vi "read_pelletronV1.vi"(8 "error in (no error)":errorcluster, 10 "Lower Timestamp Limit":i64, 11 "Upper Timestamp Limit":i64=3) -> (0 "error out":errorcluster, 3 "Array":T1[](array[typedef]))   [LabVIEW 2012]
uses:
  Pelletron.ctl
  <vilib>/addons/database/Auxilliary.llb/DB Tools Cursor Type.ctl
  <vilib>/addons/database/Connection.llb/Conn Execute.vi
  <vilib>/addons/database/Recordset.llb/Rec Fetch Recordset Data (R).vi
  <vilib>/addons/database/Recordset.llb/Rec Destroy - Connection.vi
  <vilib>/addons/database/_DB Variant To Data/Database Variant To Data.xnode
  <vilib>/addons/database/NI_Database_API.lvlib
panel:
  out "size(s)":i32
  out "SQL Query Sintax":string
  # "Pelletron"
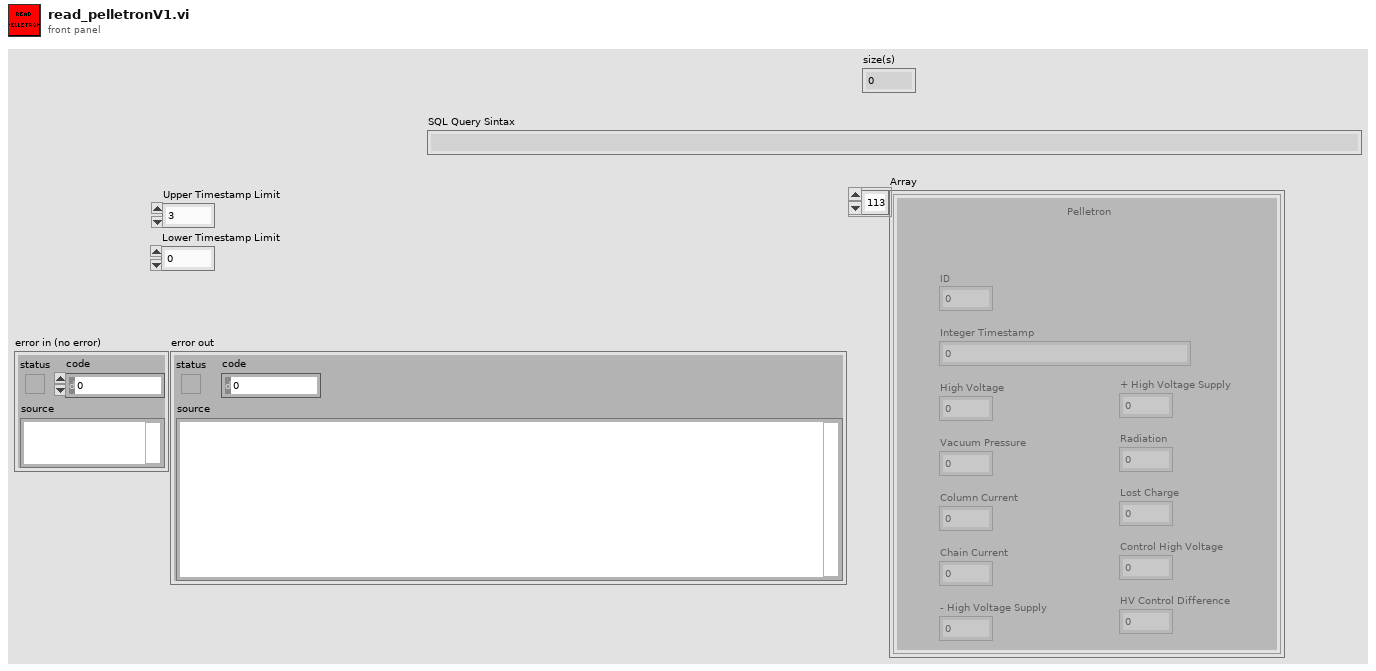
[diagram p1: front panel]
types:
  T1 = typedef "Pelletron.ctl" = cluster{"ID":i32, "Integer Timestamp":u64, "High Voltage":sgl, "+ High Voltage Supply":sgl, "- High Voltage Supply":sgl, "HV Control Difference":sgl, "Vacuum Pressure":sgl, "Radiation":sgl, "Column Current":sgl, "Lost Charge":sgl, "Chain Current":sgl, "Control High Voltage":sgl}
  T2 = typedef "NI_Database_API.lvlib/DB Tools Cursor Type.ctl" = enum16{"forward-only", "keyset", "dynamic", "static"}
  T3 = typedef "NI_Database_API.lvlib/Conn ObjectReference.ctl" = refnum<k1>
  T4 = typedef "NI_Database_API.lvlib/Rec ObjectReference.ctl" = refnum<k1>
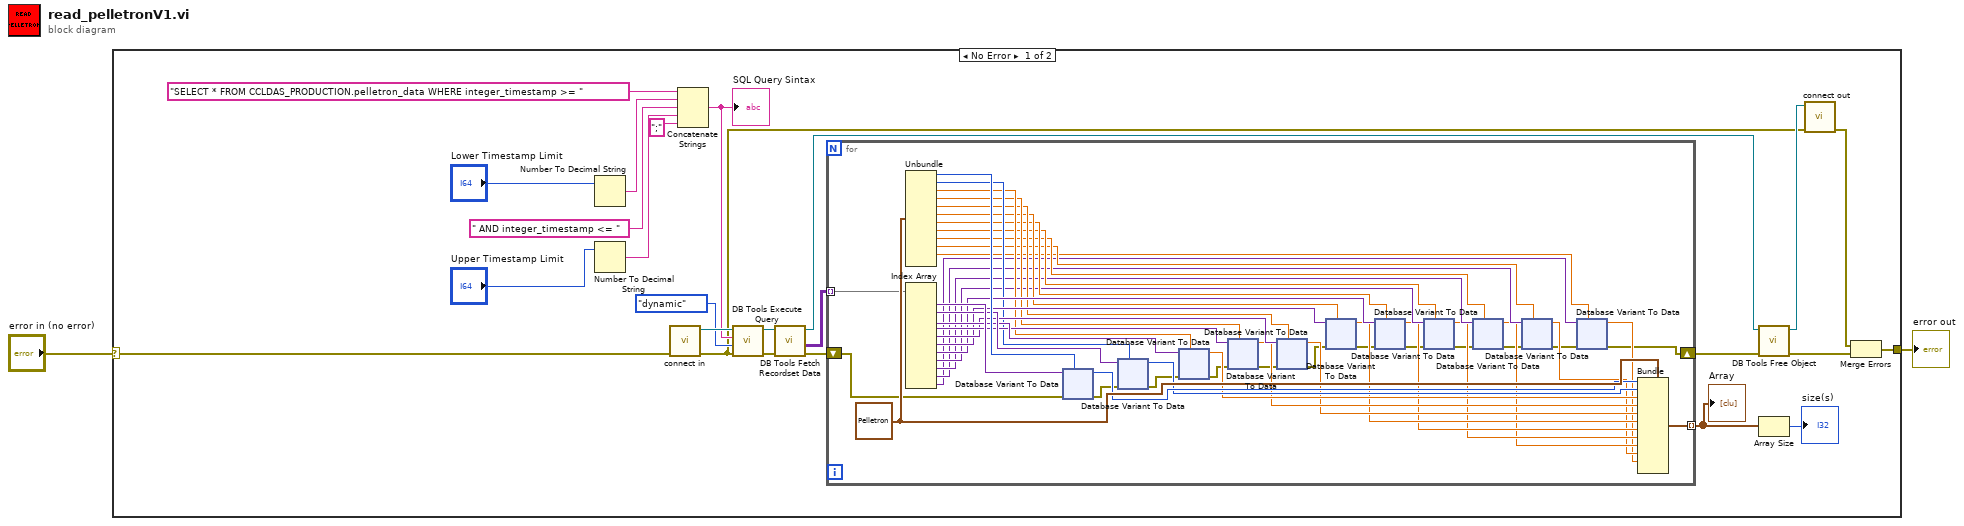
[diagram p0: block diagram]
diagram:
  n1 = case shown="No Error" "error in (no error)" {
    selector: "error in (no error)" -> [w26 w427]
    tunnel: [w5 w427] -> w1
    frame No Error {
      n2 = Number To Decimal String(number="Lower Timestamp Limit") -> (decimal integer string=w14:string)  [unwired: 1 in]
      n3 = Number To Decimal String(number="Upper Timestamp Limit") -> (decimal integer string=w11:string)  [unwired: 1 in]
      n4 = call "connect in.vi"("error in (no error)"=w26) -> ("error out"=w3:errorcluster, "Database Connection"=w20:T3)  [unwired: 6 in, 1 out]
      n5 = Concatenate Strings("SELECT * FROM CCLDAS_PRODUCTION.pelletron_data WHERE integer_timestamp >= " ("string"), w14, " AND integer_timestamp <= " ("string"), w11, ";" ("string")) -> (w19:string)
      "SQL Query Sintax" <- w19
      n6 = call-poly <vilib>:"DB Tools Execute Query.vi"("error in (no error)"=w3, "cursor type"=DB_Tools_Cursor_Type."dynamic", "SQL query"=w19, "connection reference"=w20) -> ("error out"=w16:errorcluster, "recordset reference"=w17:T4)  [unwired: 4 in]
      n7 = call-poly <vilib>:"DB Tools Fetch Recordset Data.vi"("error in (no error)"=w16, "recordset reference"=w17) -> ("error out"=w12:errorcluster, "recordset data"=w13:variant[][], "recordset reference out"=w10:T4)  [unwired: 3 in]
      n8 = for {
        tunnel: w13 -> [w73] mode=indexing
        tunnel: [w29] -> w8 mode=indexing
        shift-right: [w27] -> w9
        shift-left: w12 -> [w28]
        w74 = T1 {"ID"=0, "Integer Timestamp"=0, "High Voltage"=0.0, "+ High Voltage Supply"=0.0, "- High Voltage Supply"=0.0, "HV Control Difference"=0.0, "Vacuum Pressure"=0.0, "Radiation"=0.0, "Column Current"=0.0, "Lost Charge"=0.0, "Chain Current"=0.0, "Control High Voltage"=0.0} ("Cluster")
        n9 = Unbundle(w74) -> ("ID"=w72:i32, "Integer Timestamp"=w62:u64, "High Voltage"=w61:sgl, "+ High Voltage Supply"=w60:sgl, "- High Voltage Supply"=w59:sgl, "HV Control Difference"=w58:sgl, "Vacuum Pressure"=w57:sgl, "Radiation"=w56:sgl, "Column Current"=w55:sgl, "Lost Charge"=w54:sgl, "Chain Current"=w53:sgl)  [unwired: 1 out]
        n10 = Index Array(array=w73) -> (element #1=w70:variant, element #2=w69:variant, element #3=w68:variant, element #4=w67:variant, element #5=w66:variant, element #6=w65:variant, element #7=w64:variant, element #8=w52:variant, element #9=w51:variant, element #10=w50:variant, element #11=w49:variant)  [unwired: 11 in]
        n11 = xnode "Database Variant To Data"("database variant"=w70, "error in (no error)"=w28, "type"=w72) -> ("data"=w71:i32, "error out"=w39:errorcluster)
        n12 = xnode "Database Variant To Data"("database variant"=w69, "error in (no error)"=w39, "type"=w62) -> ("data"=w63:u64, "error out"=w38:errorcluster)
        n13 = xnode "Database Variant To Data"("database variant"=w68, "error in (no error)"=w38, "type"=w61) -> ("data"=w48:sgl, "error out"=w37:errorcluster)
        n14 = xnode "Database Variant To Data"("database variant"=w67, "error in (no error)"=w37, "type"=w60) -> ("data"=w47:sgl, "error out"=w36:errorcluster)
        n15 = xnode "Database Variant To Data"("database variant"=w66, "error in (no error)"=w36, "type"=w59) -> ("data"=w46:sgl, "error out"=w35:errorcluster)
        n16 = xnode "Database Variant To Data"("database variant"=w65, "error in"=w35, "type"=w58) -> ("data"=w45:sgl, "error out"=w34:errorcluster)
        n17 = xnode "Database Variant To Data"("database variant"=w64, "error in (no error)"=w34, "type"=w57) -> ("data"=w44:sgl, "error out"=w33:errorcluster)
        n18 = xnode "Database Variant To Data"("database variant"=w52, "error in"=w33, "type"=w56) -> ("data"=w43:sgl, "error out"=w32:errorcluster)
        n19 = xnode "Database Variant To Data"("database variant"=w51, "error in (no error)"=w32, "type"=w55) -> ("data"=w42:sgl, "error out"=w31:errorcluster)
        n20 = xnode "Database Variant To Data"("database variant"=w50, "error in"=w31, "type"=w54) -> ("data"=w41:sgl, "error out"=w30:errorcluster)
        n21 = xnode "Database Variant To Data"("database variant"=w49, "error in (no error)"=w30, "type"=w53) -> ("data"=w40:sgl, "error out"=w27:errorcluster)
        n22 = Bundle(cluster=w74, "ID"=w71, "Integer Timestamp"=w63, "High Voltage"=w48, "+ High Voltage Supply"=w47, "- High Voltage Supply"=w46, "HV Control Difference"=w45, "Vacuum Pressure"=w44, "Radiation"=w43, "Column Current"=w42, "Lost Charge"=w41, "Chain Current"=w40) -> (w29:T1)  [unwired: 1 in]
      }
      "Array" <- w8
      n23 = call-poly <vilib>:"DB Tools Free Object.vi"("error in (no error)"=w9, "recordset reference"=w10) -> ("error out"=w4:errorcluster, "connection reference"=w15:T3)  [unwired: 8 in]
      n24 = Array Size(array=w8) -> (size(s)=→"size(s)":i32)
      n25 = call "connect out.vi"("error in (no error)"=w3, "connection reference"=w15) -> ("error out"=w6:errorcluster)  [unwired: 9 in]
      n26 = Merge Errors(w6, w4) -> (w5:errorcluster)
    }
    frame Error {
    }
  }
  "error out" <- w1
